vi "Transaction.vi"(6 "Bytes to Read (100)":u32=100, 7 "Address":u16, 8 "error in (no error)":errorcluster, 9 "Parameter in":u8[](array[numeric]), 10 "Command":string, 11 "VISA Resource in":refnum<visa-resource-name>) -> (0 "error out":errorcluster, 1 "Parameter out":u8[](array[numeric]), 3 "VISA Resource out":refnum<visa-resource-name>)   [LabVIEW 2015, in "KIT QV.lvlib"]
doc: "This VI handles the low level comminication with the device. It also checks the instrument response for error conditions. Error information is inserted into the error out."
uses:
  KIT QV.lvlib
panel:
  out "read buffer":string
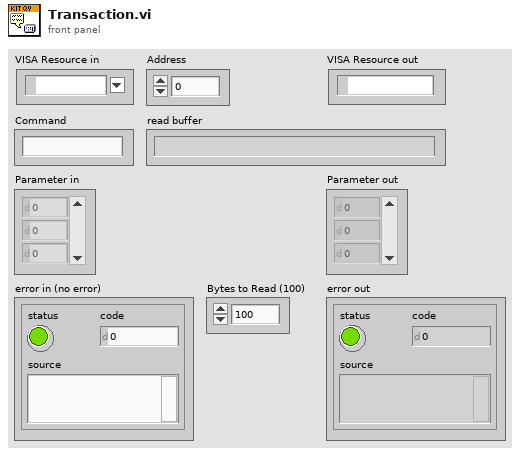
[diagram p1: front panel]
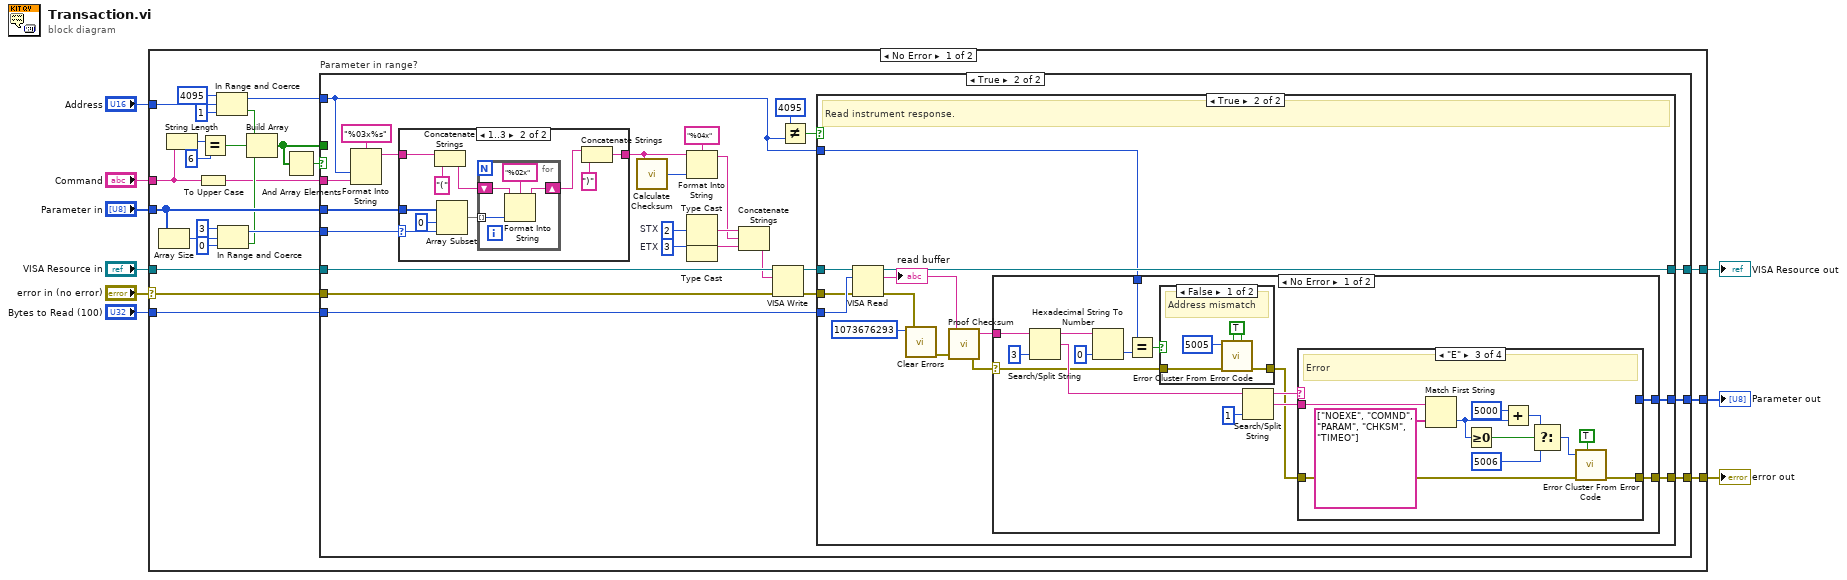
[diagram p0: block diagram]
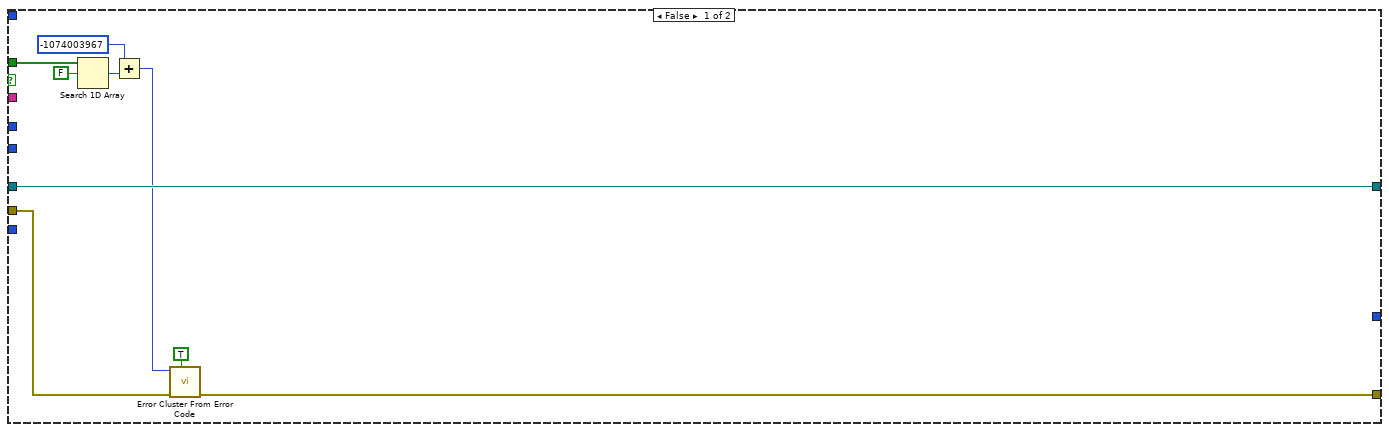
[diagram p2: hidden frame]
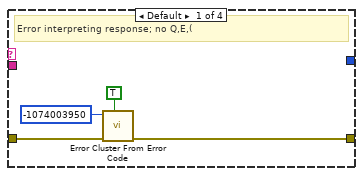
[diagram p5: hidden frame]
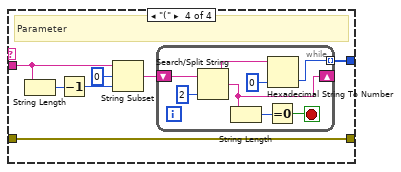
[diagram p7: hidden frame]
diagram:
  n1 = case shown="No Error" "error in (no error)" {
    selector: "error in (no error)" -> [w30 w150]
    tunnel: [w24 w150] -> w1
    tunnel: [w33 w151] -> w9
    tunnel: "Command" -> [w21 _]
    tunnel: "Bytes to Read (100)" -> [w32 _]
    tunnel: "VISA Resource in" -> [w31 w151]
    tunnel: "Address" -> [w13 _]
    tunnel: "Parameter in" -> [w29 _]
    tunnel: [w23 _] -> w2
    frame No Error {
      n2 = Array Size(array=w29) -> (size(s)=w28:i32)
      n3 = String Length(string=w21) -> (length=w20:i32)
      n4 = To Upper Case(1:w21) -> (0:w17:string)
      n5 = Equal?(x=w20, y=6) -> (x = y?=w18:bool)
      n6 = In Range and Coerce(upper limit=u16 4095 ("y"), x=w13, lower limit=u16 1) -> (coerced(x)=w12:u16, In Range?=w14:bool)
      n7 = In Range and Coerce(upper limit=3, x=w28, lower limit=0) -> (coerced(x)=w25:i32, In Range?=w22:bool)
      n8 = Build Array(w14, w18, w22) -> (w15:bool[])
      n9 = And Array Elements(Boolean array=w15) -> (logical AND=w16:bool)
      n10 = case "Parameter in range?" shown="True" w16 {
        tunnel: [w42 w67] -> w33
        tunnel: w32 -> [_ w66]
        tunnel: w31 -> [w42 w65]
        tunnel: w17 -> [_ w60]
        tunnel: w30 -> [w41 w59]
        tunnel: w29 -> [_ w57]
        tunnel: w25 -> [_ w56]
        tunnel: w12 -> [_ w45]
        tunnel: [w39 w49] -> w24
        tunnel: [_ w48] -> w23
        tunnel: w15 -> [w38 _]
        frame False {
          n11 = Search 1D Array(1D array=w38, element=FALSE) -> (index of element=w35:i32)  [unwired: 1 in]
          n12 = Add(x=-1074003967, y=w35) -> (x+y=w34:i32)
          n13 = call <vilib>:"Error Cluster From Error Code.vi"("show call chain? (False)"=TRUE, "error in (no error)"=w41, "error code (0)"=w34) -> ("error out"=w39:errorcluster)  [unwired: 6 in]
        }
        frame True {
          w62 = u8 3  # ETX
          w63 = u8 2  # STX
          n14 = Format Into String(format string="%03x%s", w45, w60) -> (resulting string=w55:string)  [unwired: 2 in, 1 out]
          n15 = case shown="1..3" w56 {
            selector: w56 -> [_ w144]
            tunnel: w57 -> [_ w145]
            tunnel: w55 -> [w135 w141]
            tunnel: [w135 w136] -> w53
            frame 0, Default {
            }
            frame 1..3 {
              n16 = Concatenate Strings(w141, "(" ("initial string")) -> (w139:string)
              n17 = Array Subset(array=w145, index=0, length=w144) -> (w142:u8[])
              n18 = for {
                tunnel: w142 -> [w148] mode=indexing
                shift-right: [w146] -> w137
                shift-left: w139 -> [w149]
                n19 = Format Into String(format string="%02x", initial string=w149, w148) -> (resulting string=w146:string)  [unwired: 1 in, 1 out]
              }
              n20 = Concatenate Strings(w137, ")" ("initial string")) -> (w136:string)
            }
          }
          n21 = call "Calculate Checksum.vi"("String in"=w53) -> ("Checksum"=w51:u16)
          n22 = Format Into String(format string="%04x", initial string=w53, w51) -> (resulting string=w52:string)  [unwired: 1 in, 1 out]
          n23 = Type Cast(x=w63) -> (*(type *) &x=w54:string)  [unwired: 1 in]
          n24 = Type Cast(x=w62) -> (*(type *) &x=w61:string)  [unwired: 1 in]
          n25 = Concatenate Strings(w54, w52, w61) -> (w64:string)
          n26 = VISA Write(VISA resource name=w65, write buffer=w64, error in (no error)=w59) -> (VISA resource name out=w46:refnum<visa-resource-name>, error out=w47:errorcluster)  [unwired: 1 out]
          n27 = Not Equal?(x=u16 4095 ("y"), y=w45) -> (x != y?=w43:bool)
          n28 = case shown="True" w43 {
            tunnel: [w69 w82] -> w67
            tunnel: w66 -> [_ w81]
            tunnel: [w68 w77] -> w49
            tunnel: [_ w76] -> w48
            tunnel: w47 -> [w68 w75]
            tunnel: w46 -> [w69 w74]
            tunnel: w45 -> [_ w73]
            frame False {
              # "Broadcast, no response expected!"
            }
            frame True {
              # "Read instrument response."
              n29 = VISA Read(VISA resource name=w74, byte count=w81, error in (no error)=w75) -> (VISA resource name out=w82:refnum<visa-resource-name>, read buffer=w80:string, error out=w72:errorcluster)  [unwired: 1 out]
              "read buffer" <- w80
              n30 = call <vilib>:"Clear Errors.vi"("error in (no error)"=w72, "specific error code to clear (0: all)"=1073676293) -> ("error out"=w71:errorcluster)  [unwired: 4 in, 1 out]
              n31 = call "Proof Checksum.vi"("Error In"=w71, "Read Buffer"=w80) -> ("Error Out"=w78:errorcluster, "Response"=w79:string)  [unwired: 1 in, 1 out]
              n32 = case shown="No Error" w78 {
                selector: w78 -> [w85 w134]
                tunnel: w79 -> [w97 _]
                tunnel: w73 -> [w92 _]
                tunnel: [w87 w134] -> w77
                tunnel: [w86 _] -> w76
                frame No Error {
                  n33 = Search/Split String(string=w97, offset (0)=3) -> (substring before match=w95:string, match + rest of string=w91:string)  [unwired: 1 in, 1 out]
                  n34 = Hexadecimal String To Number(string=w95, default (0uL)=u16 0 ("input 1")) -> (number=w93:u16)  [unwired: 1 in, 1 out]
                  n35 = Equal? ("Check address")(x=w92, y=w93) -> (x = y?=w83:bool)
                  n36 = case shown="False" w83 {
                    tunnel: w85 -> [w101 w102]
                    tunnel: [w100 w102] -> w84
                    frame False {
                      w99 = TRUE ("show call chain? (False)")
                      # "Address mismatch"
                      n37 = call <vilib>:"Error Cluster From Error Code.vi"("is warning? (False)"=w99, "show call chain? (False)"=w99, "error in (no error)"=w101, "error code (0)"=5005) -> ("error out"=w100:errorcluster)  [unwired: 5 in]
                    }
                    frame True {
                      # "Address OK"
                    }
                  }
                  n38 = Search/Split String(string=w91, offset (0)=1 ("length (rest)")) -> (substring before match=w89:string, match + rest of string=w88:string)  [unwired: 1 in, 1 out]
                  n39 = case shown="\"E\"" w89 {
                    tunnel: w88 -> [_ _ w117 w124]
                    tunnel: w84 -> [w104 w107 w116 w119]
                    tunnel: [w103 w107 w113 w119] -> w87
                    tunnel: [_ _ _ w120] -> w86
                    frame Default {
                      # "Error interpreting response; no Q,E,("
                      n40 = call <vilib>:"Error Cluster From Error Code.vi"("show call chain? (False)"=TRUE, "error in (no error)"=w104, "error code (0)"=-1074003950) -> ("error out"=w103:errorcluster)  [unwired: 6 in]
                    }
                    frame "Q" {
                      # "Acknowledge"
                    }
                    frame "E" {
                      # "Error"
                      n41 = Match First String(2:string[] ["NOEXE", "COMND", "PARAM", "CHKSM", "TIMEO"] ("string array"), 3:w117) -> (0:w112:i32)  [unwired: 1 out]
                      n42 = Greater Or Equal To 0?(x=w112) -> (x >= 0?=w111:bool)
                      n43 = Add(x=5000, y=w112) -> (x+y=w110:i32)
                      n44 = Select(t=w110, s=w111, f=5006) -> (s? t:f=w109:i32)
                      n45 = call <vilib>:"Error Cluster From Error Code.vi"("show call chain? (False)"=TRUE, "error in (no error)"=w116, "error code (0)"=w109) -> ("error out"=w113:errorcluster)  [unwired: 6 in]
                    }
                    frame "(" {
                      # "Parameter"
                      n46 = String Length(string=w124) -> (length=w125:i32)
                      n47 = Decrement(x=w125) -> (x-1=w123:i32)
                      n48 = String Subset(string=w124, offset (0)=0, length (rest)=w123) -> (substring=w121:string)
                      n49 = while {
                        shift-right: [w128] -> _
                        shift-left: w121 -> [w133]
                        tunnel: [w126] -> w120 mode=indexing
                        stop <- w131 stop-if-true
                        n50 = Search/Split String(string=w133, offset (0)=2) -> (substring before match=w129:string, match + rest of string=w128:string)  [unwired: 1 in, 1 out]
                        n51 = String Length(string=w128) -> (length=w130:i32)
                        n52 = Equal To 0?(x=w130) -> (x = 0?=w131:bool)
                        n53 = Hexadecimal String To Number(string=w129, default (0uL)=u8 0 ("default (0 U32)")) -> (number=w126:u8)  [unwired: 1 in, 1 out]
                      }
                    }
                  }
                }
                frame Error {
                }
              }
            }
          }
        }
      }
    }
    frame Error {
    }
  }
  "error out" <- w1
  "VISA Resource out" <- w9
  "Parameter out" <- w2
